vi "Vert_Spread_2_Sig.vi"(1 "Index":i32) -> (0 "resulting string":string)   [LabVIEW 2010]
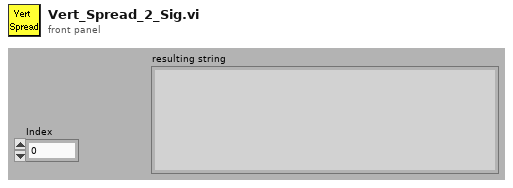
[diagram p1: front panel]
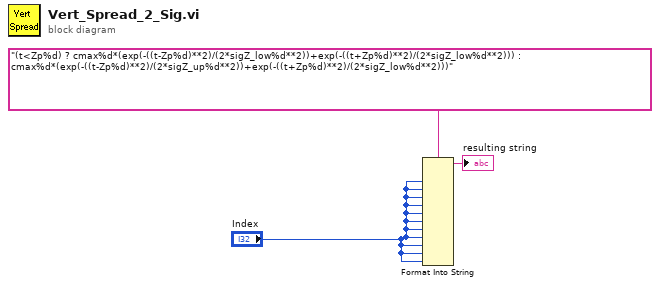
[diagram p0: block diagram]
diagram:
  n1 = Format Into String(format string="(t<Zp%d) ? cmax%d*(exp(-((t-Zp%d)**2)/(2*sigZ_low%d**2))+exp(-((t+Zp%d)**2)/(2*sigZ_low%d**2))) : cmax%d*(exp(-((t-Zp%d)**2)/(2*sigZ_up%d**2))+exp(-((t+Zp%d)**2)/(2*sigZ_low%d**2)))", "Index", "Index", "Index", "Index", "Index", "Index", "Index", "Index", "Index", "Index", "Index") -> (resulting string=→"resulting string":string)  [unwired: 2 in, 1 out]
